vi "Interpret_Tag.vi"(9 "byte order":T1(ring)=enum."little-endian", 11 "String in":string) -> (0 "text translated":string, 2 "Tag":T3, 3 "String out":string)   [LabVIEW 2022 SP3]
uses:
  miDataType.ctl
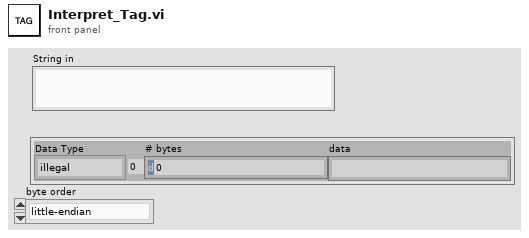
[diagram p1: front panel]
types:
  T1 = enum16{"big-endian, network order", "native, host order", "little-endian"}
  T2 = typedef "miDataType.ctl" = enum16{"illegal", "miINT8", "miUINT8", "miINT16", "miUINT16", "miINT32", "miUINT32", "miSINGLE", "--", "miDOUBLE", "---", "----", "miINT64", "miUINT64", "miMATRIX", "miCOMPRESSED", "miUTF8", "miUTF16", "miUTF32", "udefined"}
  T3 = cluster{"Data Type":T2, "# bytes":u32, "data":string}
  T4 = cluster{"Value":u32, "Value":u32, "String out":string}
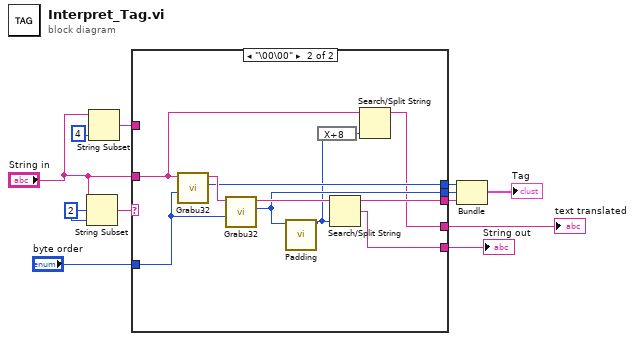
[diagram p0: block diagram]
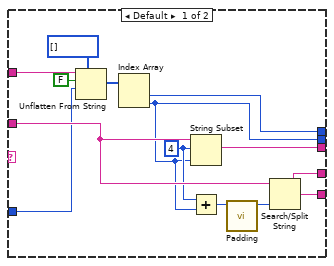
[diagram p2: hidden frame]
diagram:
  w7 = 2 ("offset (0)")
  n1 = String Subset(string="String in", offset (0)=w7, length (rest)=w7) -> (substring=w6:string)
  n2 = String Subset(string="String in", length (rest)=4 ("offset (0)")) -> (substring=w3:string)  [unwired: 1 in]
  n3 = case shown="\"\\00\\00\"" w6 {
    tunnel: [w22 w37] -> w11
    tunnel: [w19 w36] -> w10
    tunnel: [w18 w33] -> w9
    tunnel: [w14 w32] -> w8
    tunnel: "String in" -> [w21 w30]
    tunnel: w3 -> [w24 _]
    tunnel: "byte order" -> [w15 w31]
    tunnel: [w13 w29] -> w1
    frame Default {
      w20 = 4 ("offset (0)")
      n4 = Unflatten From String(type=u16[] [], binary string=w24, data includes array or string size? (T)=FALSE, byte order (0:big-endian, network order)=w15) -> (value=w23:u16[])  [unwired: 1 in, 2 out]
      n5 = Index Array(array=w23) -> (element #1=w18:u16, element #2=w14:u16)  [unwired: 2 in]
      n6 = String Subset(string=w21, offset (0)=w20, length (rest)=w14) -> (substring=w22:string)
      n7 = Add(x=w20, y=w14) -> (x+y=w16:i32)
      n8 = call "Padding.vi"("bytes in"=w16) -> ("total bytes"=w17:i32)  [unwired: 9 in, 1 out]
      n9 = Search/Split String(string=w21, offset (0)=w17) -> (substring before match=w13:string, match + rest of string=w19:string)  [unwired: 1 in, 1 out]
    }
    frame "\u0000\u0000\u0000" {
      n10 = call "Grabu32.vi"("byte order"=w31, "String in"=w30) -> ("Value"=w33:u32, "String out"=w34:string)  [unwired: 8 in]
      n11 = call "Grabu32.vi"("byte order"=w31, "String in"=w34) -> ("Value"=w32:u32, "String out"=w35:string)  [unwired: 8 in]
      n12 = call "Padding.vi"("bytes in"=w32) -> ("total bytes"=w27:i32)  [unwired: 9 in, 1 out]
      n13 = expression code="X+8"(w27) -> (w28:i32)
      n14 = Search/Split String(string=w35, offset (0)=w27) -> (substring before match=w37:string, match + rest of string=w36:string)  [unwired: 1 in, 1 out]
      n15 = Search/Split String(string=w30, offset (0)=w28) -> (substring before match=w29:string)  [unwired: 1 in, 2 out]
    }
  }
  "String out" <- w10
  "text translated" <- w1
  n16 = Bundle("Value"=w9, "Value"=w8, "String out"=w11) -> (→"Tag":T4)  [unwired: 1 in]
